vi "Caraya.vi"   [LabVIEW 2020]
uses:
  <vilib>/addons/_JKI Toolkits/Caraya/classes/Assert/Assert Equal Value_Variant.vi
  Libraries/Osciloscope/Osciloscope.lvlib
  <vilib>/addons/_JKI Toolkits/Caraya/classes/Test/Test.lvclass
  <vilib>/addons/_JKI Toolkits/Caraya/classes/Assert/Assert.lvclass
types:
  T1 = typedef "Osciloscope.lvlib/Broadcast Events--cluster.ctl" = cluster{"Module Did Init":refnum<user-event>, "Status Updated":refnum<user-event>, "Error Reported":refnum<user-event>, "Module Did Stop":refnum<user-event>, "Update Module Execution Status":refnum<user-event>, "Obtain Osciloscope Name":refnum<user-event>}
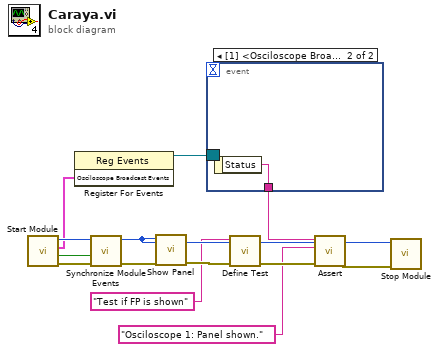
[diagram p0: block diagram]
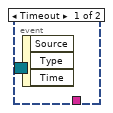
[diagram p2: hidden frame]
diagram:
  n1 = call "Start Module.vi"() -> ("error out"=w12:errorcluster, "Wait for Event Sync?"=w11:bool, "Osciloscope Broadcast Events"=w3:T1, "Module ID"=w13:i32)  [unwired: 8 in]
  n2 = register-events(w3) -> (reference out=w2:refnum<event-registration>)  [unwired: 2 in, 1 out]
  n3 = call "Synchronize Module Events.vi"("error in"=w12, "Wait for Event Sync?"=w11, "Module ID in"=w13) -> ("error out"=w10:errorcluster, "Module ID out"=w6:i32)  [unwired: 7 in]
  n4 = call "Show Panel.vi"("error in (no error)"=w10, "Module ID"=w6) -> ("error out"=w8:errorcluster)  [unwired: 9 in]
  n5 = event shown="[1] <Osciloscope Broadcast Events.Status Updated>: User Event" {
    selector: w2 -> [_ _]
    dyn-events: _ -> [_ _]
    timeout: _ -> [_ _]
    tunnel: [_ w14] -> w1
    event Timeout {
      n6 = event-data() -> ()  [unwired: 1 in, 3 out]
    }
    event User Event {
      n7 = event-data() -> ("Status"=w14:string)  [unwired: 1 in]
    }
  }
  n8 = call <vilib>:"Define Test.vi"("error in (no error)"=w8, "Label (VI Title)"="Test if FP is shown") -> ("error out"=w9:errorcluster)  [unwired: 9 in]
  n9 = call-poly <vilib>:"Assert.vi"("error in (no error)"=w9, "Y"="Osciloscope 1: Panel shown.", "X"=w1) -> ("error out"=w7:errorcluster)  [unwired: 8 in]
  n10 = call "Stop Module.vi"("error in (no error)"=w7, "Module ID"=w6) -> ()  [unwired: 9 in, 1 out]
